vi "large_histogram.vi"() -> ()   [LabVIEW 2012]
doc: "SciScan 1.2 160630"
panel:
  out "Histogram 2":T1(graph)={"Starting Value"=-2007.0, "Incremental Value"=15.7109375, "Histogram"=[]}
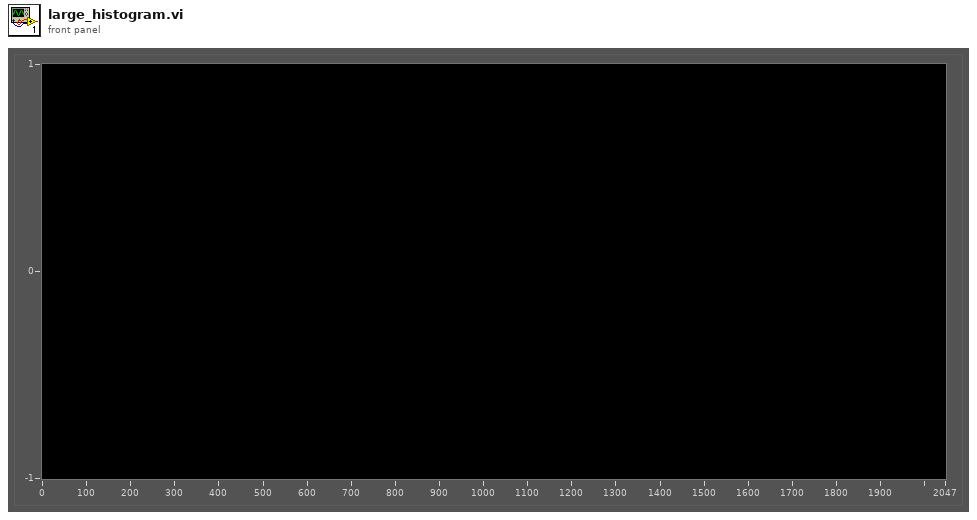
[diagram p1: front panel]
types:
  T1 = cluster{"Starting Value":sgl, "Incremental Value":sgl, "Histogram":u32[]}
  T2 = cluster{"Histogram Graph":cluster{"Starting Value":sgl, "Incremental Value":sgl, "Histogram":u32[]}, i32, i32}
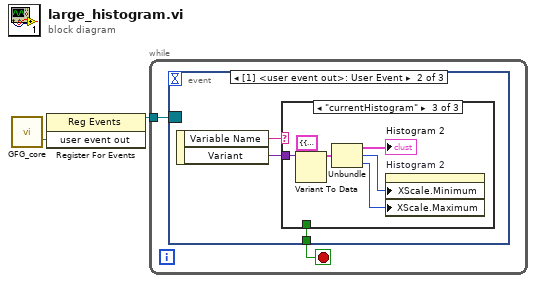
[diagram p0: block diagram]
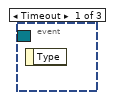
[diagram p2: hidden frame]
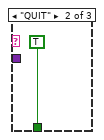
[diagram p4: hidden frame]
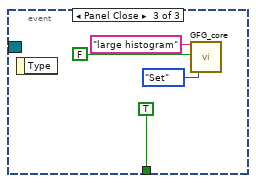
[diagram p5: hidden frame]
diagram:
  n1 = call "GFG_core.vi"() -> ("user event out"=w1:refnum<user-event>)  [unwired: 13 in, 6 out]
  n2 = register-events(w1) -> (reference out=w2:refnum<event-registration>)  [unwired: 2 in, 1 out]
  n3 = while {
    tunnel: w2 -> [w4]
    stop <- w3 stop-if-true
    n4 = event shown="[1] <user event out>: User Event" {
      selector: w4 -> [_ _ _]
      dyn-events: _ -> [_ _ _]
      timeout: _ -> [_ _ _]
      tunnel: [_ w6 TRUE] -> w3
      event Timeout {
        n5 = event-data() -> ()  [unwired: 1 in, 1 out]
      }
      event User Event {
        n6 = event-data() -> ("Variable Name"=w5:string, "Variant"=w7:variant)  [unwired: 1 in]
        n7 = case shown="\"currentHistogram\"" w5 {
          tunnel: w7 -> [_ _ w14]
          tunnel: [_ TRUE _] -> w6
          frame Default {
          }
          frame "QUIT" {
          }
          frame "currentHistogram" {
            n8 = Variant To Data(type=T2 {"Histogram Graph"={"Starting Value"=0.0, "Incremental Value"=0.0, "Histogram"=[]}, 0, 0} ("cluster"), Variant=w14) -> (data=w12:T2)  [unwired: 1 in, 1 out]
            n9 = Unbundle(w12) -> ("Histogram Graph"=→"Histogram 2":T1, w11:i32, w10:i32)
            n10 = property on="Histogram 2" class="WFGraph (strict)"("XScale.Minimum"=w11, "XScale.Maximum"=w10) -> ()  [unwired: 2 in, 2 out]
          }
        }
      }
      event Panel Close {
        n11 = event-data() -> ()  [unwired: 1 in, 1 out]
        n12 = call "GFG_core.vi"("Variable Name in"="large histogram", "Variant in"=FALSE, "Action"=enum16{"Init", "Set", "Get", "Clear"}."Set") -> ()  [unwired: 10 in, 7 out]
      }
    }
  }
